vi "DirectTF.vi"(8 "Int. Step (ms)":dbl=0.05, 9 "Action u(t)":dbl=-3.172970085949789, 10 "State Space Coeff y(t)":dbl[](array[numeric])=[5.264, 2.2833, 0.1211], 11 "State Space Coeff x1_dot(t)":dbl[](array[numeric])=[-6.5407, -3.1492]) -> (3 "NonDelayed Output":dbl)   [LabVIEW 2016]
doc: "Integration by Euler Rule Order 2 of the State Space representation of the transfer funtion of the non Foloccular visual path and eye plant. Hirata et al. 2002 Annals of the New York Academy of Sciences."
panel:
  # "State Space Representation"
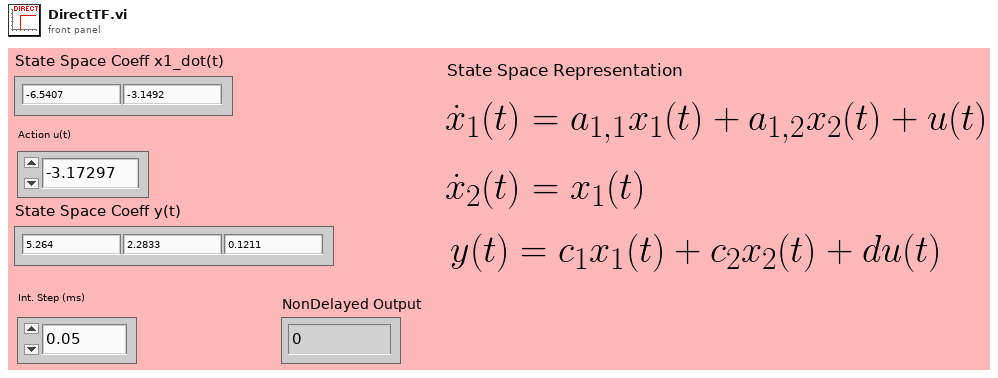
[diagram p1: front panel]
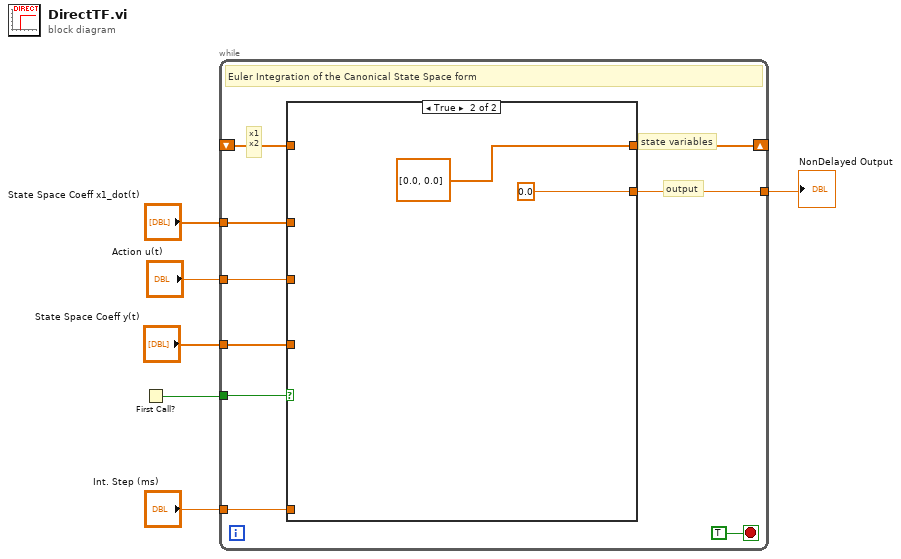
[diagram p0: block diagram]
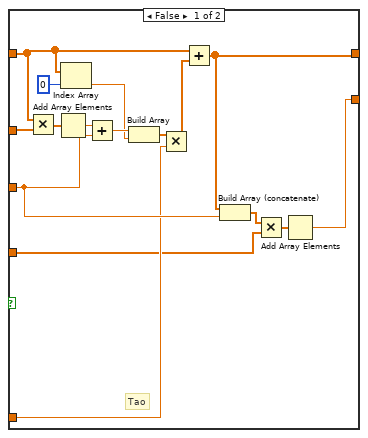
[diagram p2: hidden frame]
diagram:
  n1 = First Call?() -> (First Call?: T/F=w1:bool)
  n2 = while {
    shift-right: [w11] -> _
    shift-left: _ -> [w12]
    tunnel: w1 -> [w15]
    tunnel: "State Space Coeff x1_dot(t)" -> [w13]
    tunnel: "Int. Step (ms)" -> [w10]
    tunnel: "Action u(t)" -> [w9]
    tunnel: "State Space Coeff y(t)" -> [w8]
    tunnel: [w7] -> w2
    stop <- TRUE stop-if-true
    # "x1\nx2"
    # "output"
    # "state variables"
    # "Euler Integration of the Canonical State Space form"
    n3 = case shown="True" w15 {
      tunnel: w13 -> [w29 _]
      tunnel: w12 -> [w19 _]
      tunnel: [w17 dbl[] [0.0, 0.0]] -> w11
      tunnel: w10 -> [w25 _]
      tunnel: w9 -> [w28 _]
      tunnel: w8 -> [w20 _]
      tunnel: [w16 0.0] -> w7
      frame False {
        # "Tao"
        n4 = Multiply(x=w19, y=w29) -> (x*y=w31:dbl[])
        n5 = Add Array Elements(numeric array=w31) -> (sum=w30:dbl)
        n6 = Index Array(array=w19, index=0) -> (element=w21:dbl)
        n7 = Add(x=w30, y=w28) -> (x+y=w23:dbl)
        n8 = Build Array(w23, w21) -> (w24:dbl[])
        n9 = Multiply(x=w24, y=w25) -> (x*y=w18:dbl[])
        n10 = Add(x=w19, y=w18) -> (x+y=w17:dbl[])
        n11 = Build Array (concatenate)(w17, w28) -> (w27:dbl[])
        n12 = Multiply(x=w27, y=w20) -> (x*y=w26:dbl[])
        n13 = Add Array Elements(numeric array=w26) -> (sum=w16:dbl)
      }
      frame True {
      }
    }
  }
  "NonDelayed Output" <- w2
